vi "I2CDecode.vi"(11 "String":string) -> (1 "NofBytes":u8, 2 "Address":u8, 3 "I2CData":u8[](array[numeric]))   [LabVIEW 2017]
panel:
  out "StringOut":string
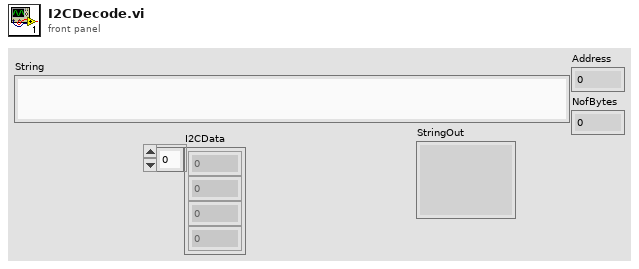
[diagram p1: front panel]
types:
  T1 = cluster{"String":string, "String":string, "String":string}
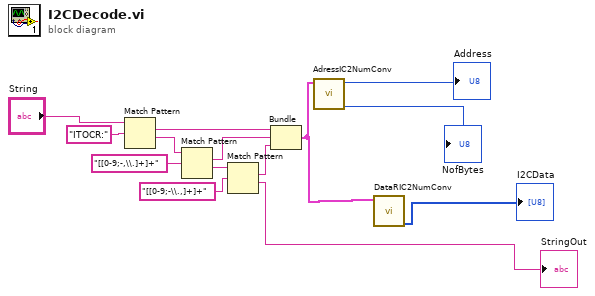
[diagram p0: block diagram]
diagram:
  n1 = Match Pattern(string="String", regular expression="ITOCR:") -> (match substring=w8:string, after substring=w12:string)  [unwired: 1 in, 2 out]
  n2 = Match Pattern(string=w12, regular expression="[[0-9;-,\\.]+]+") -> (match substring=w6:string, after substring=w9:string)  [unwired: 1 in, 2 out]
  n3 = Match Pattern(string=w9, regular expression="[[0-9;-\\.,]+]+") -> (match substring=w7:string, after substring=→"StringOut":string)  [unwired: 1 in, 2 out]
  n4 = Bundle("String"=w8, "String"=w6, "String"=w7) -> (w3:T1)  [unwired: 1 in]
  n5 = call "AdressIC2NumConv.vi"("Cluster"=w3) -> ("NofBytes"=→"NofBytes":u8, "Address"=→"Address":u8)  [unwired: 9 in]
  n6 = call "DataRIC2NumConv.vi"("Cluster"=w3) -> ("Data"=→"I2CData":u8[])  [unwired: 9 in, 1 out]
